vi "Scan Setup.vi"(8 "error in (no error)":errorcluster, 11 "Scanner in":refnum<class "Scanner.lvclass">) -> (0 "error out":errorcluster, 3 "Scanner out":refnum<class "Scanner.lvclass">)   [LabVIEW 2023, in "Scanner.lvclass"]
doc: "Configure the Instrument based on the class member fields. This step comes after the user has closed the \"Scan Setup\" window and before the actual scan -- so instruments are configured with the user's specified settings."
uses:
  Scanner.lvclass
  Scanner.lvclass/Scanner.ctl
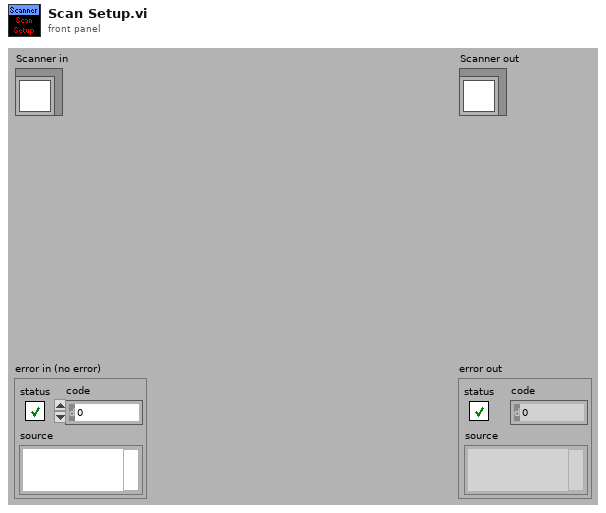
[diagram p1: front panel]
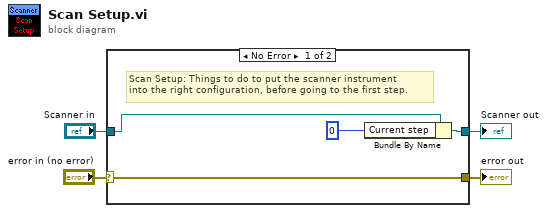
[diagram p0: block diagram]
diagram:
  n1 = case shown="No Error" "error in (no error)" {
    selector: "error in (no error)" -> [w8 w10]
    tunnel: [w8 w10] -> w3
    tunnel: [w6 w9] -> w1
    tunnel: "Scanner in" -> [w7 w9]
    frame No Error {
      # "Scan Setup: Things to do to put the scanner instrument\ninto the right configuration, before going to the first step."
      n2 = Bundle By Name(cluster=w7, "Current step"=u32 0) -> (w6:refnum<class "Scanner.lvclass">)
    }
    frame Error {
    }
  }
  "error out" <- w3
  "Scanner out" <- w1
